vi "libssh2_session_abstract.vi"(8 "error in (no error)":errorcluster, 11 "session":T2) -> (0 "error out":errorcluster, 2 "abstract":T1)   [LabVIEW 2017, in "libssh2.lvlib"]
doc: "Get the abstract data that was provided to <B>libssh2_session_init_ex</B> when creating a session."
uses:
  libssh2.lvlib
  Session Refnum.ctl
  libssh2_session_abstract.ctl
  lvssh2_session_callback_events.ctl
  lvssh2_session_callback_send_function_input_args_32.ctl
  lvssh2_session_callback_receive_function_input_args_32.ctl
  lvssh2_userauth_keyboard_interactive_response_function_input_args_32.ctl
  lvssh2_session_callback_send_function_input_args_64.ctl
  lvssh2_session_callback_receive_function_input_args_64.ctl
  lvssh2_userauth_keyboard_interactive_response_function_input_args_64.ctl
  Not A Session.vi
  <vilib>/Utility/error.llb/Error Cluster From Error Code.vi
  Global Settings.vi
  Read Session Refnum.vi
  <vilib>/Utility/semaphor.llb/Acquire Semaphore.vi
  <vilib>/Utility/semaphor.llb/Release Semaphore.vi
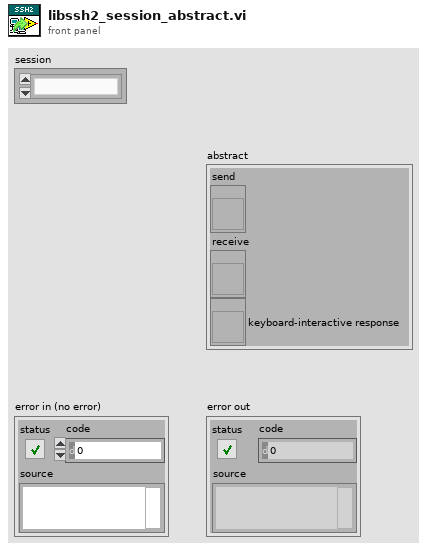
[diagram p1: front panel]
types:
  T1 = typedef "libssh2.lvlib/libssh2_session_abstract.ctl" = cluster{"send":refnum<vi>, "receive":refnum<vi>, "keyboard-interactive response":refnum<vi>}
  T2 = typedef "libssh2.lvlib/Session Refnum.ctl" = refnum<k1>
  T3 = typedef "libssh2.lvlib/lvssh2_session_callback_events.ctl" = cluster{"32-bit":cluster{"send":refnum<user-event>, "recv":refnum<user-event>, "kbdint_response":refnum<user-event>}, "64-bit":cluster{"send":refnum<user-event>, "recv":refnum<user-event>, "kbdint_response":refnum<user-event>}, "stop":cluster{"send":refnum<user-event>, "recv":refnum<user-event>, "kbdint_response":refnum<user-event>}}
  T4 = cluster{"send":refnum<user-event>, "recv":refnum<user-event>, "kbdint_response":refnum<user-event>}
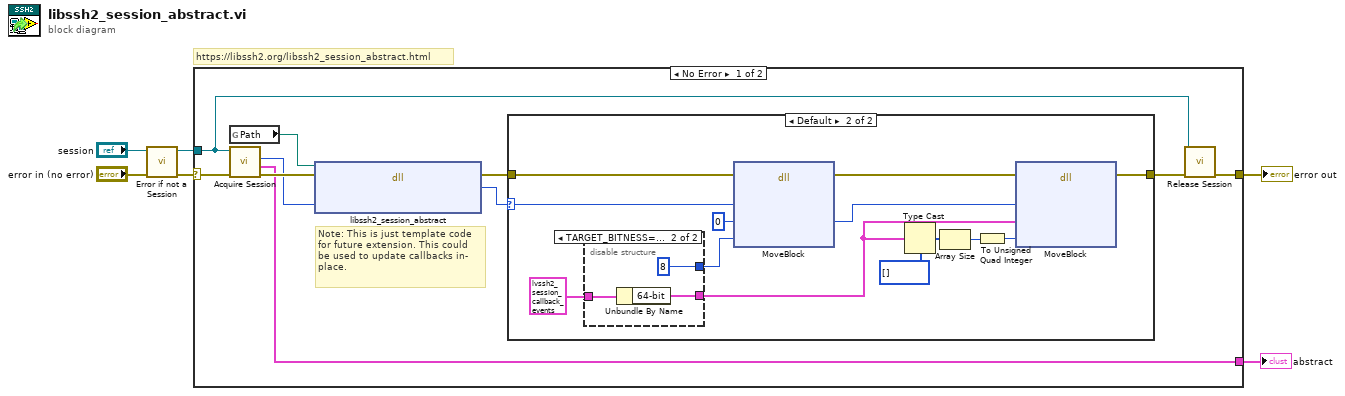
[diagram p0: block diagram]
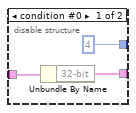
[diagram p3: hidden frame]
diagram:
  # "https://libssh2.org/libssh2_session_abstract.html"
  n1 = call "Error if not a Session.vi"("error in (no error)"="error in (no error)", "session"="session") -> ("error out"=w4:errorcluster, "session out"=w2:T2)  [unwired: 8 in]
  n2 = case shown="No Error" w4 {
    selector: w4 -> [w7 w37]
    tunnel: [w9 w37] -> w6
    tunnel: w2 -> [w8 _]
    tunnel: [w10 _] -> w1
    frame No Error {
      # "Note: This is just template code\nfor future extension. This could\nbe used to update callbacks in-\nplace."
      n3 = global read "Global Settings.vi" "Path"() -> (w14:path)
      n4 = call "Acquire Session.vi"("error in (no error)"=w7, "session"=w8) -> ("error out"=w16:errorcluster, "abstract"=w10:T1, "LIBSSH2_SESSION*"=w15:u64)  [unwired: 7 in]
      n5 = dll-call lib="?" fn="libssh2_session_abstract"(path in=w14, error in=w16, "session"=w15) -> (error out=w13:errorcluster, "return value"=w11:u64)  [unwired: 2 in, 1 out]
      n6 = case shown="Default" w11 {
        selector: w11 -> [_ w23]
        tunnel: w13 -> [w17 w24]
        tunnel: [w17 w30] -> w12
        frame 0 {
        }
        frame Default {
          n7 = disable-structure shown="TARGET_BITNESS==64" {
            disable-tunnel: T3 {"32-bit"={"send"=refnum, "recv"=refnum, "kbdint_response"=refnum}, "64-bit"={"send"=refnum, "recv"=refnum, "kbdint_response"=refnum}, "stop"={"send"=refnum, "recv"=refnum, "kbdint_response"=refnum}} ("events") -> [w33 w36]
            disable-tunnel: [w32 w35] -> w25
            disable-tunnel: [u64 4 ("size") u64 8 ("size")] -> w18
            frame condition #0 {
              n8 = Unbundle By Name(w33) -> ("32-bit"=w32:T4)
            }
            frame condition #1 (active) {
              n9 = Unbundle By Name(w36) -> ("64-bit"=w35:T4)
            }
          }
          n10 = dll-call lib="LabVIEW" fn="MoveBlock"(error in=w24, "ps"=w23, "pd"=u64 0, "size"=w18) -> (error out=w21:errorcluster, "pd"=w20:u64)  [unwired: 5 in, 1 out]
          n11 = Type Cast(type=u8[] [], x=w25) -> (*(type *) &x=w28:u8[])
          n12 = Array Size(array=w28) -> (size(s)=w27:i32)
          n13 = To Unsigned Quad Integer(1:w27) -> (0:w26:u64)
          n14 = dll-call lib="LabVIEW" fn="MoveBlock"(error in=w21, "ps"=w20, "pd"=w25, "size"=w26) -> (error out=w30:errorcluster)  [unwired: 6 in, 1 out]
        }
      }
      n15 = call "Release Session.vi"("error in (no error)"=w12, "session"=w8) -> ("error out"=w9:errorcluster)  [unwired: 9 in]
    }
    frame Error {
    }
  }
  "error out" <- w6
  "abstract" <- w1
